vi "Build Map.vi"(4 "Goal":T1, 5 "Walls":cluster{"Y":dbl, "X":dbl}[](array[cluster]), 6 "Objects bottom cords":T3(array[cluster]), 7 "Robot":cluster{"Y":dbl, "X":dbl, "Bearing":dbl}) -> (0 "GoalPoint":T1, 1 "Updated Corners":cluster{"Col":dbl, "Row":dbl}[](array[cluster]), 2 "Updated Map":T2, 3 "Robot in map":cluster{"Col":dbl, "Row":dbl})   [LabVIEW 2009]
uses:
  <vilib>/Analysis/Matrix/Datatypes/RealMatrix.ctl
  ControlProject/Drive/Drive_Point.ctl
  <vilib>/Analysis/Matrix/NI_Matrix.lvlib
  ControlProject/Drive.lvlib
panel:
  in  "Robot cluster":cluster{"Col":dbl, "Row":dbl}
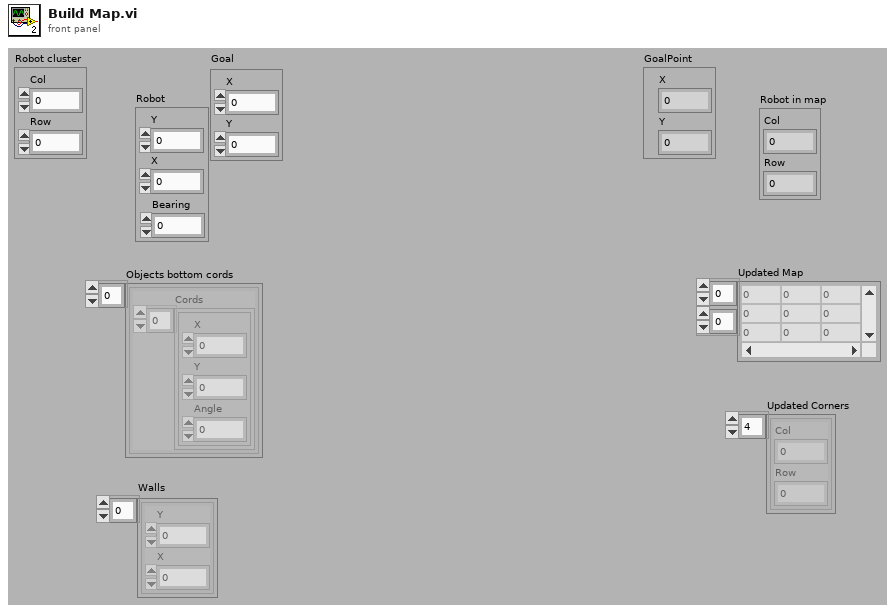
[diagram p1: front panel]
types:
  T1 = typedef "Drive.lvlib/Drive_Point.ctl" = cluster{"X":dbl, "Y":dbl}
  T2 = typedef "NI_Matrix.lvlib/RealMatrix.ctl" = dbl[][]
  T3 = cluster{"Cords":cluster{"X":dbl, "Y":dbl, "Angle":dbl}[]}[]
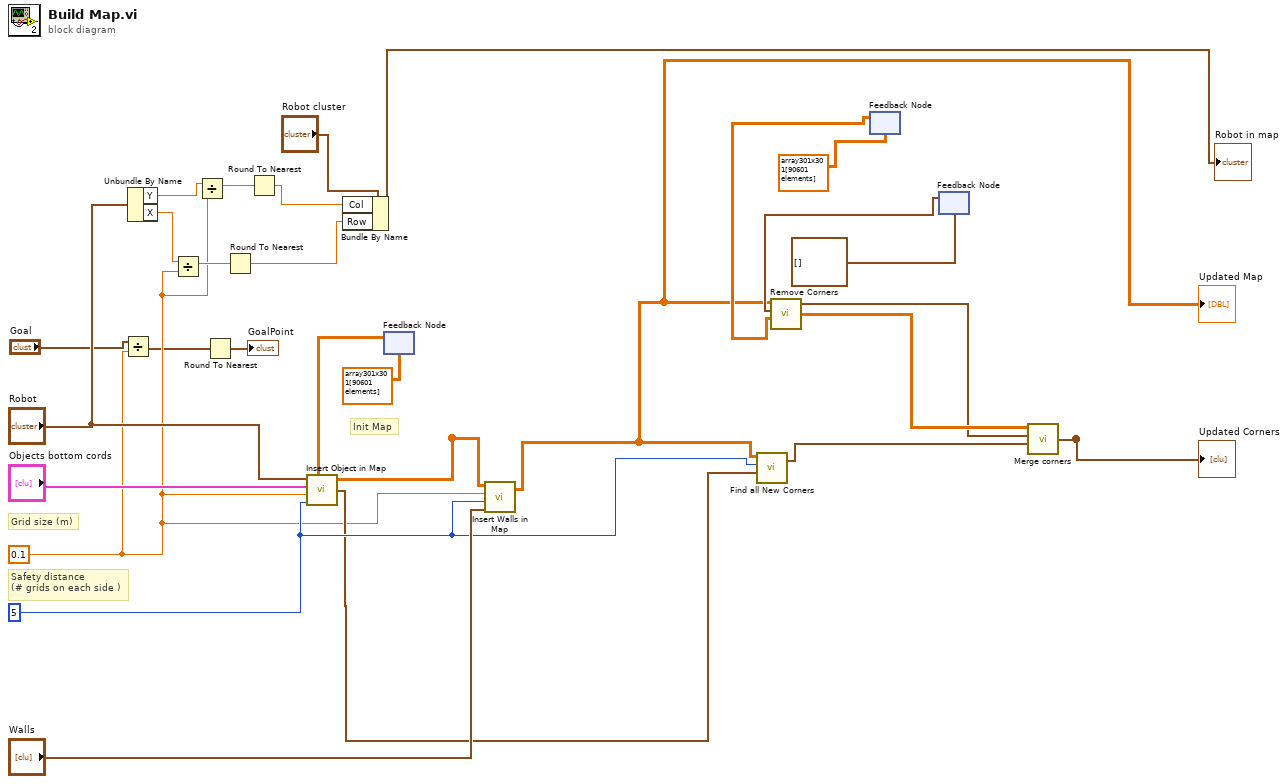
[diagram p0: block diagram]
diagram:
  w16 = 5
  w3 = 0.1
  # "Init Map"
  # "Safety distance \n(# grids on each side )"
  # "Grid size (m)"
  n1 = Divide(x="Goal", y=w3) -> (x/y=w2:T1)
  n2 = Unbundle By Name("Robot") -> ("Y"=w9:dbl, "X"=w11:dbl)
  n3 = Divide(x=w11, y=w3) -> (x/y=w13:dbl)
  n4 = Divide(x=w9, y=w3) -> (x/y=w10:dbl)
  n5 = Round To Nearest(number=w2) -> (nearest integer value=→"GoalPoint":T1)
  n6 = Round To Nearest(number=w13) -> (nearest integer value=w5:dbl)
  n7 = Round To Nearest(number=w10) -> (nearest integer value=w6:dbl)
  n8 = Bundle By Name(cluster="Robot cluster", "Col"=w6, "Row"=w5) -> (→"Robot in map":cluster{"Col":dbl, "Row":dbl})
  n9 = feedback #1(T2 array301x301[90601 elements] ("matrix")) -> (w20:T2)
  n10 = call "Insert Object in Map.vi"("Robot"="Robot", "Map"=w20, "Objects bottom cords"="Objects bottom cords", "Grid size (m)"=w3, "# safety grids"=w16) -> ("Updated Map"=w18:T2, "Points"=w15:cluster{"Col":dbl, "Row":dbl}[])  [unwired: 2 in]
  n11 = call "Insert Walls in Map.vi"("Map"=w18, "Grid size"=w3, "# safety grids"=w16, "Walls"="Walls") -> ("Updated Map"=w17:T2)  [unwired: 2 in]
  "Updated Map" <- w17
  n12 = call "Find all New Corners.vi"("Points"=w15, "# safety grids"=w16, "Updated Map"=w17) -> ("Corners"=w14:cluster{"Col":dbl, "Row":dbl}[])  [unwired: 2 in]
  n13 = feedback #2(T2 array301x301[90601 elements] ("Updated Corners Matrix")) -> (w27:T2)
  n14 = feedback #3(cluster{"Col":dbl, "Row":dbl}[] [] ("New old corners")) -> (w24:cluster{"Col":dbl, "Row":dbl}[])
  n15 = call "Remove Corners.vi"("Old Corners Matrix"=w27, "Old corners"=w24, "Updated Map"=w17) -> ("Updated Corners Matrix"=w30:T2, "New old corners"=w29:cluster{"Col":dbl, "Row":dbl}[])  [unwired: 2 in]
  n16 = call "Merge corners.vi"("New Corners"=w14, "Old corners"=w29, "Corners Matrix"=w30) -> ("Updated Corners"=w25:cluster{"Col":dbl, "Row":dbl}[], "Updated Corners Matrix"=w28:T2)  [unwired: 2 in]
  "Updated Corners" <- w25
